vi "getStringBounds.vi"(0 "reference":refnum<class "Graphics.lvclass">, 1 "text":string, 2 "fontType":T2, 3 "font":T3, 5 "error in (no error)":errorcluster) -> (14 "reference out":refnum<class "Graphics.lvclass">, 15 "bounds":T1 {"height" format="%.2f"; "width" format="%.2f"; "y" format="%.2f"; "x" format="%.2f"}, 19 "error out":errorcluster)   [LabVIEW 2012, in "Graphics.lvclass"]
doc: "Gets the size of a string"
uses:
  <resource>/Framework/Providers/Open_GDS/UML/Graphics_class/Graphics.lvclass
  <resource>/Framework/Providers/Open_GDS/UML/Graphics_class/FontType.ctl
  <resource>/Framework/Providers/Open_GDS/UML/Graphics_class/LvFontType.ctl
  <resource>/Framework/Providers/Open_GDS/UML/General/Rectangle/Rectangle Rectangle2D.ctl
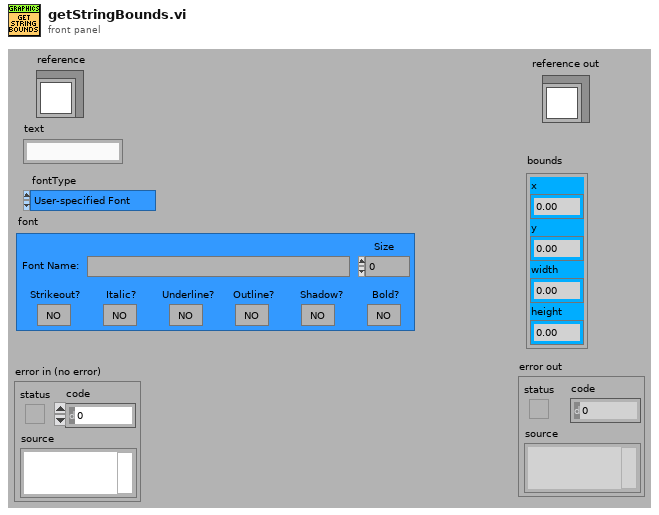
[diagram p1: front panel]
types:
  T1 = typedef "Rectangle Rectangle2D.ctl" = cluster{"x":dbl, "y":dbl, "width":dbl, "height":dbl}
  T2 = typedef "Graphics.lvclass/LvFontType.ctl" = enum16{"User-specified Font", "Application Font", "System Font", "Dialog Font"}
  T3 = typedef "Graphics.lvclass/FontType.ctl" = cluster{"Font Name:":string, "Size":i16, "Strikeout?":bool, "Italic?":bool, "Underline?":bool, "Outline?":bool, "Shadow?":bool, "Bold?":bool}
  T4 = cluster{"left":i16, "top":i16, "right":i16, "bottom":i16}
  T5 = typedef "Graphics.lvclass/ObjectAttributes.ctl" = cluster{"drawColor":u32, "backgroundColor":u32, "font":T3, "fontType":T2, "picture":picture, "stroke":T6, "scaleX":dbl, "scaleY":dbl, "screenRef":refnum<vi>, "offsetX":dbl, "offsetY":dbl}
  T6 = typedef "Graphics.lvclass/StrokeType.ctl" = enum16{"USE_DEFAULT", "SOLID", "DOTTED"}
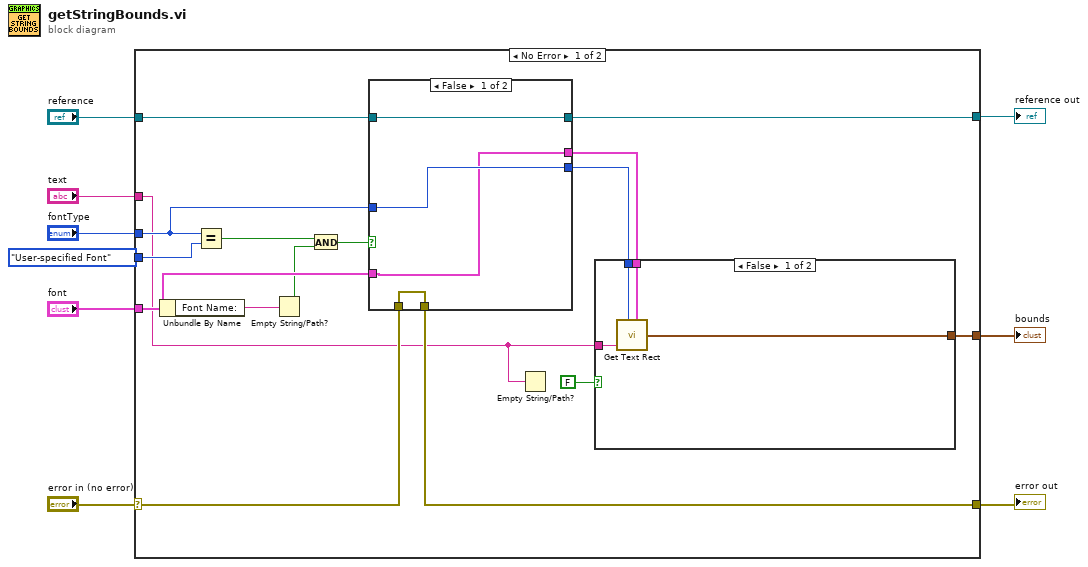
[diagram p0: block diagram]
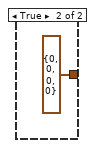
[diagram p2: hidden frame]
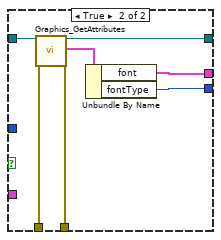
[diagram p3: hidden frame]
diagram:
  n1 = case shown="No Error" "error in (no error)" {
    selector: "error in (no error)" -> [w13 w42]
    tunnel: "reference" -> [w15 w43]
    tunnel: [w12 w42] -> w7
    tunnel: [w14 w43] -> w6
    tunnel: "fontType" -> [w19 _]
    tunnel: LvFontType."User-specified Font" ("fontType") -> [w25 _]
    tunnel: "font" -> [w24 _]
    tunnel: "text" -> [w11 _]
    tunnel: [w16 _] -> w1
    frame No Error {
      n2 = Unbundle By Name(w24) -> ("Font Name:"=w23:string)
      n3 = Equal?(x=w19, y=w25) -> (x = y?=w22:bool)
      n4 = Empty String/Path?(string/path=w23) -> (empty?=w21:bool)
      n5 = And(x=w22, y=w21) -> (x .and. y?=w20:bool)
      n6 = case shown="False" w20 {
        tunnel: [w34 w36] -> w18
        tunnel: [w33 w37] -> w17
        tunnel: w24 -> [w33 _]
        tunnel: w19 -> [w34 _]
        tunnel: w15 -> [w32 w41]
        tunnel: [w32 w40] -> w14
        tunnel: w13 -> [w31 w39]
        tunnel: [w31 w38] -> w12
        frame False {
        }
        frame True {
          n7 = call <resource>:"Graphics_GetAttributes.vi"("reference in"=w41, "error in (no error)"=w39) -> ("reference out"=w40:refnum<class "Graphics.lvclass">, "Data"=w35:T5, "error out"=w38:errorcluster)  [unwired: 1 in, 14 out]
          n8 = Unbundle By Name(w35) -> ("font"=w37:T3, "fontType"=w36:T2)
        }
      }
      n9 = Empty String/Path?(string/path=w11) -> ()  [unwired: 1 out]
      n10 = case shown="False" FALSE {
        tunnel: w18 -> [w29 _]
        tunnel: w17 -> [w28 _]
        tunnel: [w27 T4 {"left"=0, "top"=0, "right"=0, "bottom"=0} ("rect")] -> w16
        tunnel: w11 -> [w26 _]
        frame False {
          n11 = call <vilib>:"Get Text Rect.vi"("desired font(Application)"=w29, "text"=w26, "[user-specified font]"=w28) -> ("rect"=w27:T4)  [unwired: 3 in, 3 out]
        }
        frame True {
        }
      }
    }
    frame Error {
    }
  }
  "reference out" <- w6
  "error out" <- w7
  "bounds" <- w1
